vi "TirfModuleStep.vi"() -> ()   [LabVIEW 2012]
doc: "DESCRIPTION:\nThe One-Axis Move (Accel - Max Velocity - Decel) VI completes a move to user-specified position on a single axis while using user-specified acceleration, maximum velocity, and deceleration values. It also provides a monitor to track the progress of the move.\n\n*Note: This VI can be used as a subVI in a higher level program.\n\nINSTRUCTIONS:\n(1) Be sure your board is initialized before running this VI. Refer to the Initialization topic in the FlexMotion VI Online Help, which can be launched by choosing FlexMotion VI Online Help in the Help menu.\n\n(2) Select the Board ID that corresponds to your FlexMotion controller in the Board Configuration Utility. \n\n(3) Select the axis number to be used.\n\n(4) Set the Target Position (in encoder counts) to which you want the axis to move.\n\n(5) Set the values you wish to use for maximum velocity (RPM), acceleration (RPS/S), and deceleration (RPS/S).\n\n(6) Run the VI.\n\nKEY PARAMETERS:\n(1) Target Position: The position to which you want to move. This value needs to be changed every time you run the VI. If you run the VI twice in a row with the same target position, the motor will not move the second time since it will already be at its target position.\n\n(2) Velocity: The maximum velocity for the specified axis during the move.\n\n(3) Acceleration: The acceleration for the axis during the move.\n\n(4) Deceleration: The deceleration for the axis during the move. (This may be different than the acceleration.)\n\nI/O CONNECTIONS OVERVIEW:\nThis example requires a system configuration with one axis."
uses:
  MicroDrive.dll
panel:
  in  "Move This Axis":u16(ring)=1 items=["1"=1, "2"=2, "3"=3, "4"=4, "5"=5, "6"=6]
  out "M6 Forward Limit":bool
  out "M6 Reverse Limit":bool
  out "M5 Forward Limit":bool
  out "M5 Reverse Limit":bool
  out "M4 Forward Limit":bool
  out "M4 Reverse Limit":bool
  in  "Reset M4":bool
  in  "Flip M4 Encoder":bool
  out "M4 Encoder (um)":dbl format="%.3f"
  in  "Flip M3 Encoder":bool
  in  "Flip M2 Encoder":bool
  in  "Flip M1 Encoder":bool
  out "M3 Encoder (um)":dbl format="%.3f"
  in  "Reset M3":bool
  out "M3 Forward Limit":bool
  out "M3 Reverse Limit":bool
  out "M2 Forward Limit":bool
  out "M2 Reverse Limit":bool
  out "M1 Forward Limit":bool
  out "M1 Reverse Limit":bool
  out "M2 Encoder (um)":dbl format="%.3f"
  in  "Reset  All":bool
  in  "Reset M2":bool
  out "M1 Encoder (um)":dbl format="%.3f"
  in  "Reset M1":bool
  out "Found Epi":bool
  in  "EPI Axis":u16(ring)=6 items=["1"=1, "2"=2, "3"=3, "4"=4, "5"=5, "6"=6]
  in  "Load":bool
  in  "Save":bool
  in  "clear5":bool
  in  "clear4":bool
  in  "clear3":bool
  in  "clear2":bool
  in  "clear1":bool
  in  "clear all":bool
  in  "write 5":bool
  in  "write 4":bool
  in  "write 3":bool
  in  "write 2":bool
  in  "write 1":bool
  in  "p4":bool
  in  "p5":bool
  in  "p3":bool
  in  "p2":bool
  in  "p1":bool
  out "Cluster":cluster{"Name":string[], "Position":dbl[]}
  out "Array 2":string[](array[string])
  out "Array":dbl[](array[numeric])
  out "Moving":bool
  in  "EPI":bool
  in  "Store":bool
  out "Current Position":dbl
  in  "Direction:":bool=TRUE
  out "Device Handle":i32
  in  "Velocity (mm/s)":dbl=1.0 min=0.01 max=2.0 format="%.3f"
  in  "Move size (µm)":dbl=50.0 format="%.3f"
  out "Forward Limit":bool
  out "Reverse Limit":bool
  in  "stop":bool
  in  "Move":bool
  # "Move To:"
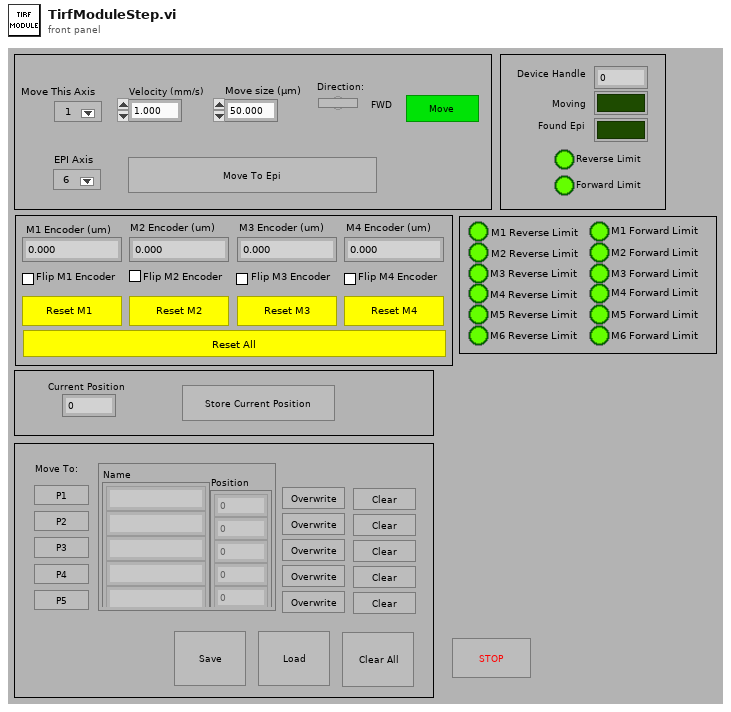
[diagram p1: front panel]
types:
  T1 = enum8{"Enabled", "Disabled", "Disabled and Grayed Out"}
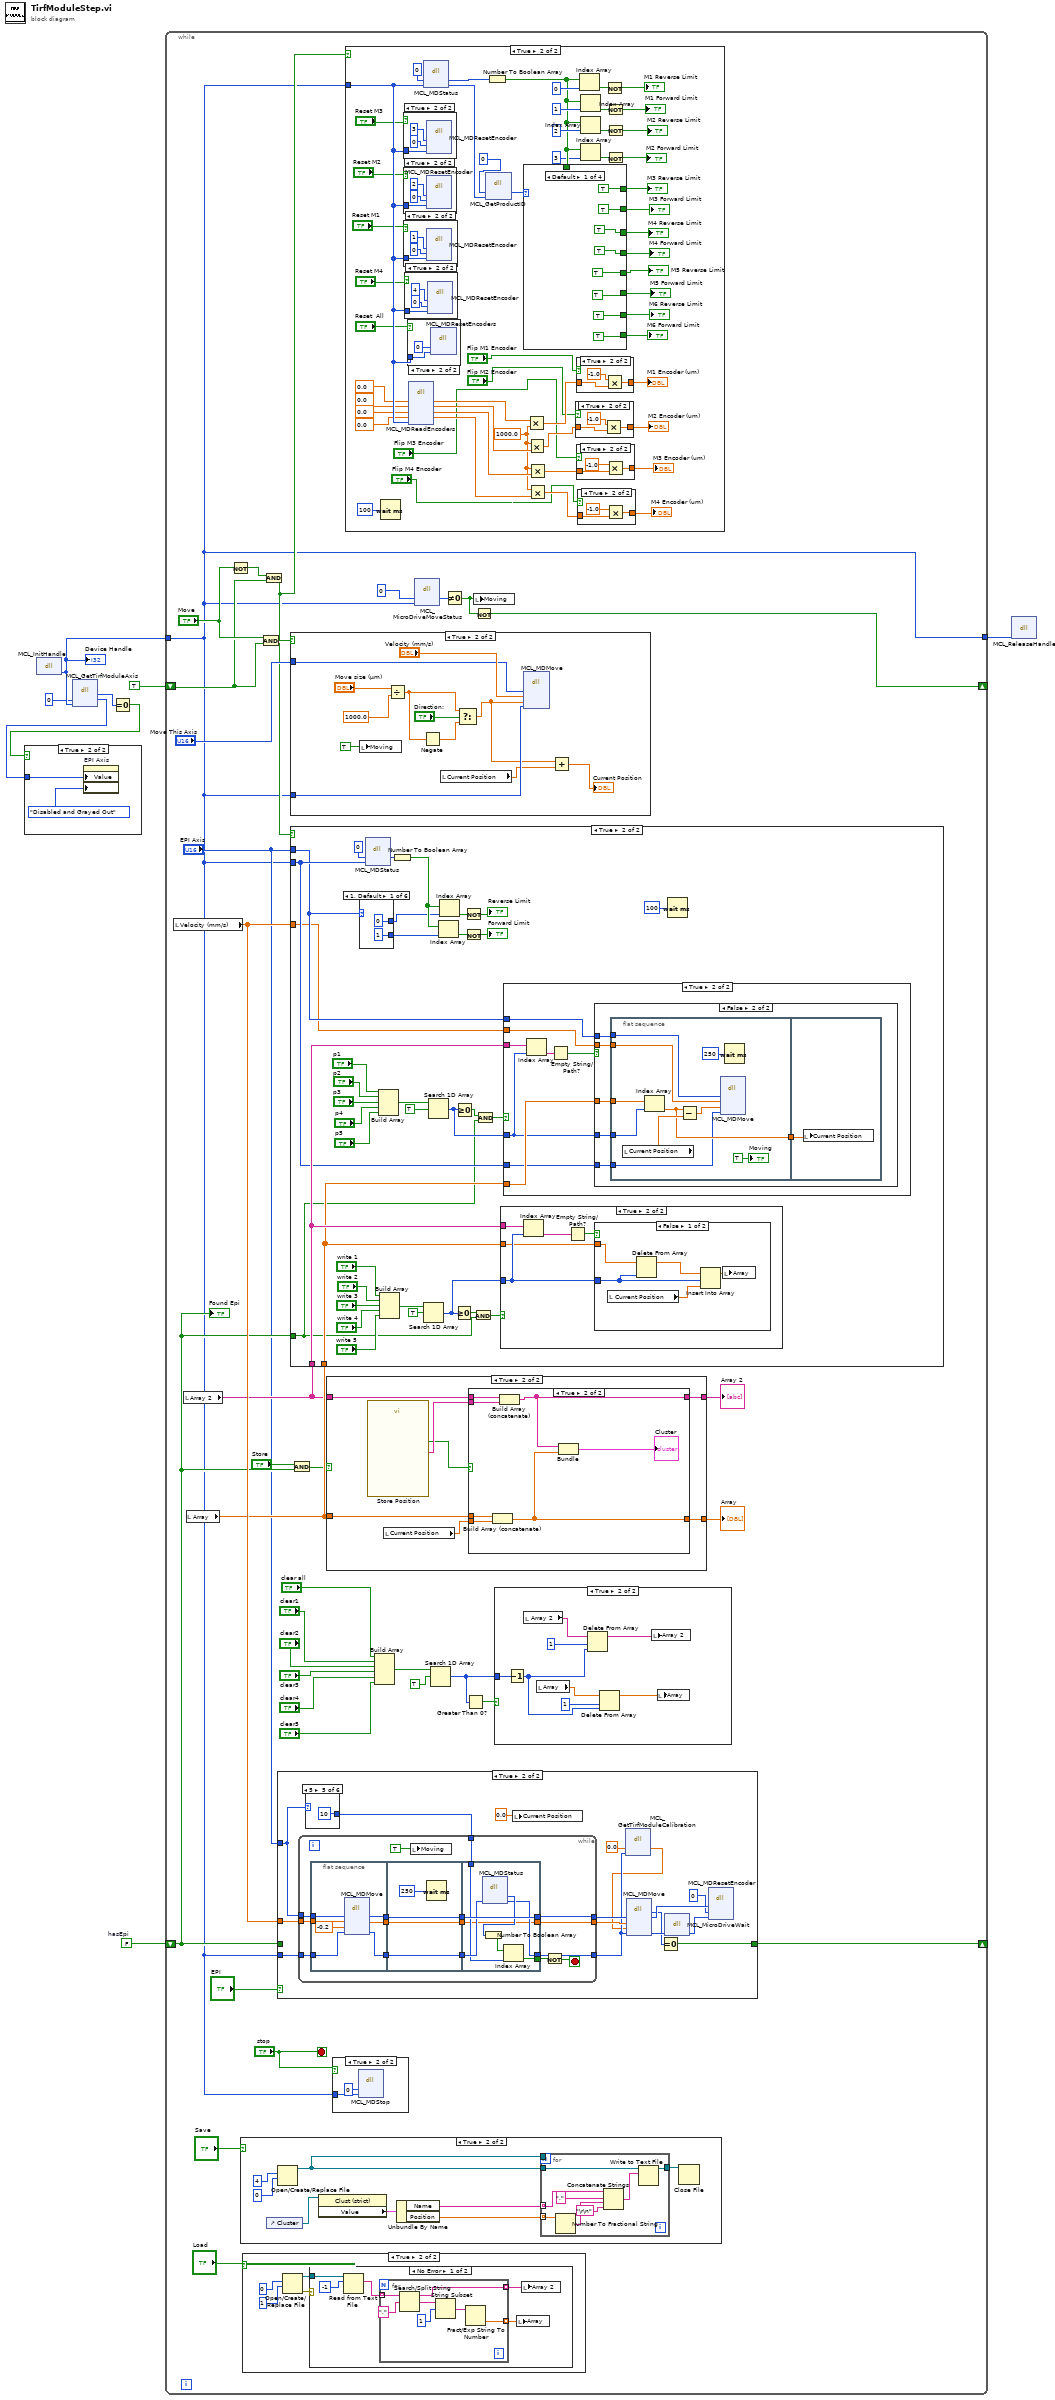
[diagram p0: block diagram]
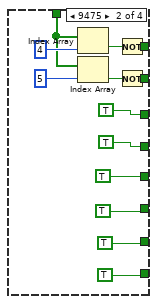
[diagram p9: hidden frame]
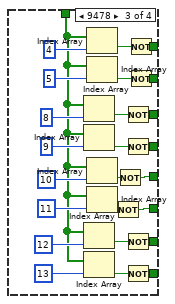
[diagram p10: hidden frame]
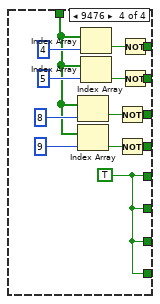
[diagram p11: hidden frame]
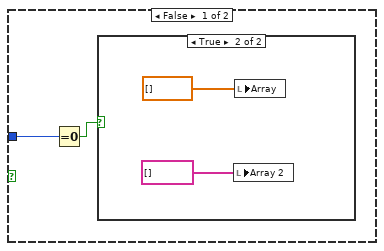
[diagram p19: hidden frame]
diagram:
  w6 = FALSE  # hasEpi
  n1 = dll-call lib="C:/Users/Labview/Desktop/TirfModuleStep/MicroDrive.dll" fn="MCL_InitHandle"() -> ("return type"=w5:i32)  [unwired: 3 in, 2 out]
  "Device Handle" <- w5
  n2 = dll-call lib="C:/Users/Labview/Desktop/TirfModuleStep/MicroDrive.dll" fn="MCL_GetTirfModuleAxis"("axis"=u16 0, "handle"=w5) -> ("return type"=w3:i32, "axis"=w1:i32)  [unwired: 4 in, 2 out]
  n3 = Equal To 0?(x=w3) -> (x = 0?=w2:bool)
  n4 = case shown="True" w2 {
    tunnel: w1 -> [_ w10]
    frame False {
    }
    frame True {
      n5 = property on="EPI Axis" class="Ring (strict)"("Value"=w10, "DisabledEnum"=T1."Disabled and Grayed Out" ("Disabled")) -> ()  [unwired: 2 in, 2 out]
    }
  }
  n6 = while {
    tunnel: w5 -> [w15]
    shift-right: [w12] -> _
    shift-left: TRUE -> [w43]
    tunnel: [w15] -> w7
    shift-right: [w22] -> _
    shift-left: w6 -> [w19]
    stop <- "stop" stop-if-true
    n7 = local read "Velocity (mm/s)"() -> (w40:dbl)
    n8 = local read "Array 2"() -> (w37:string[])
    n9 = local read "Array"() -> (w39:dbl[])
    n10 = Not(x="Move") -> (.not. x?=w44:bool)
    n11 = case shown="True" "Save" {
      frame False {
      }
      frame True {
        n12 = control-ref of="Cluster"() -> (w212:refnum<vi>)
        n13 = Open/Create/Replace File(operation (0:open)=4, access (0:read/write)=0) -> (refnum out=w206:refnum<file>)  [unwired: 4 in, 2 out]
        n14 = property class="Clust (strict)"(reference=w212) -> ("Value"=w211:cluster{"Name":string[], "Position":dbl[]})  [unwired: 1 in, 2 out]
        n15 = Unbundle By Name(w211) -> ("Name"=w207:string[], "Position"=w205:dbl[])
        n16 = for {
          tunnel: w205 -> [w219] mode=indexing
          tunnel: w206 -> [_]
          tunnel: [w220] -> w208
          tunnel: w207 -> [w214] mode=indexing
          tunnel: w206 -> [w213]
          n17 = Number To Fractional String(number=w219) -> (F-format string=w215:string)  [unwired: 3 in]
          n18 = Concatenate Strings(w214, ",", w215, "\r\n") -> (w217:string)
          n19 = Write to Text File(file (use dialog)=w213, text=w217) -> (refnum out=w220:refnum<file>)  [unwired: 2 in, 2 out]
        }
        n20 = Close File(refnum=w208) -> ()  [unwired: 1 in, 2 out]
      }
    }
    n21 = case shown="True" "Load" {
      frame False {
      }
      frame True {
        n22 = Open/Create/Replace File(operation (0:open)=0, access (0:read/write)=1) -> (refnum out=w189:refnum<file>, error out=w190:errorcluster)  [unwired: 4 in, 1 out]
        n23 = case shown="No Error" w190 {
          tunnel: w189 -> [w197 _]
          frame No Error {
            n24 = Read from Text File(file (use dialog)=w197, count=-1) -> (text=w195:string[])  [unwired: 2 in, 3 out]
            n25 = for {
              tunnel: w195 -> [w204] mode=indexing
              tunnel: [w202] -> w194 mode=indexing
              tunnel: [w198] -> w193 mode=indexing
              n26 = Search/Split String(string=w204, search string/char (-)=",") -> (substring before match=w202:string, match + rest of string=w201:string)  [unwired: 1 in, 1 out]
              n27 = String Subset(string=w201, offset (0)=1) -> (substring=w199:string)  [unwired: 1 in]
              n28 = Fract/Exp String To Number(string=w199) -> (number=w198:dbl)  [unwired: 3 in, 1 out]
            }
            n29 = local write "Array"(w193) -> ()
            n30 = local write "Array 2"(w194) -> ()
          }
          frame Error {
          }
        }
      }
    }
    n31 = And(x="Move", y=w43) -> (x .and. y?=w42:bool)
    n32 = And(x=w44, y=w43) -> (x .and. y?=w16:bool)
    n33 = case shown="True" "EPI" {
      tunnel: w40 -> [_ w334]
      tunnel: w15 -> [_ w333]
      tunnel: "EPI Axis" -> [_ w330]
      tunnel: w19 -> [w318 _]
      tunnel: [w318 w319] -> w22
      frame False {
      }
      frame True {
        n34 = case shown="5" w330 {
          tunnel: [0 2 4 8 10 12] -> w329
          frame 1, Default {
          }
          frame 2 {
          }
          frame 3 {
          }
          frame 4 {
          }
          frame 5 {
          }
          frame 6 {
          }
        }
        n35 = while {
          tunnel: w334 -> [w356]
          tunnel: w333 -> [w352]
          tunnel: [w351] -> w322
          tunnel: w330 -> [w354]
          tunnel: [w353] -> w327
          tunnel: w329 -> [w346]
          tunnel: [w342] -> w328
          stop <- w355 stop-if-true
          n36 = flat-sequence {
            tunnel: w356 -> [w363]
            tunnel: w354 -> [w361]
            tunnel: w352 -> [w359]
            tunnel: [w360] -> w350
            tunnel: [w358] -> w349
            tunnel: [w357] -> w344
            tunnel: w350 -> [w367]
            tunnel: w349 -> [w366]
            tunnel: [w367] -> w348
            tunnel: [w366] -> w347
            tunnel: w344 -> [w364]
            tunnel: [w364] -> w343
            tunnel: [w371] -> w351
            tunnel: [w375] -> w353
            tunnel: w348 -> [w375]
            tunnel: w347 -> [w372]
            tunnel: w346 -> [w370]
            tunnel: [w369] -> w345
            tunnel: w343 -> [w368]
            tunnel: [w368] -> w342
            frame #0 {
              n37 = dll-call lib="C:/Users/Labview/Desktop/TirfModuleStep/MicroDrive.dll" fn="MCL_MDMove"("axis"=w361, "velocity"=w363, "distance"=-0.2, "handle"=w359) -> ("axis"=w360:i32, "velocity"=w357:dbl, "handle"=w358:i32)  [unwired: 4 in, 3 out]
            }
            frame #1 {
              n38 = Wait (ms)(milliseconds to wait=u32 250) -> ()  [unwired: 1 out]
            }
            frame #2 {
              n39 = dll-call lib="C:/Users/Labview/Desktop/TirfModuleStep/MicroDrive.dll" fn="MCL_MDStatus"("handle"=w372) -> ("status"=w374:u16, "handle"=w371:i32)  [unwired: 3 in, 4 out]
              n40 = Number To Boolean Array(number=w374) -> (Boolean array=w373:bool[])
              n41 = Index Array(array=w373, index=w370) -> (element=w369:bool)
            }
          }
          n42 = local write "Moving"(TRUE ("is Moving")) -> ()
          n43 = Not(x=w345) -> (.not. x?=w355:bool)
        }
        n44 = local write "Current Position"(0.0) -> ()
        n45 = dll-call lib="C:/Users/Labview/Desktop/TirfModuleStep/MicroDrive.dll" fn="MCL_GetTirfModuleCalibration"("calMM"=0.0 ("distance"), "handle"=w322) -> ("calMM"=w321:dbl)  [unwired: 4 in, 3 out]
        n46 = dll-call lib="C:/Users/Labview/Desktop/TirfModuleStep/MicroDrive.dll" fn="MCL_MDMove"("axis"=w327, "velocity"=w328, "distance"=w321, "handle"=w322) -> ("return type"=w320:i32, "axis"=w325:i32, "handle"=w331:i32)  [unwired: 5 in, 2 out]
        n47 = Equal To 0?(x=w320) -> (x = 0?=w319:bool)
        n48 = dll-call lib="C:/Users/Labview/Desktop/TirfModuleStep/MicroDrive.dll" fn="MCL_MicroDriveWait"("handle"=w331) -> ("handle"=w326:i32)  [unwired: 3 in, 3 out]
        n49 = dll-call lib="C:/Users/Labview/Desktop/TirfModuleStep/MicroDrive.dll" fn="MCL_MDResetEncoder"("axis"=w325, "status"=u16 0 ("distance"), "handle"=w326) -> ()  [unwired: 5 in, 4 out]
      }
    }
    n50 = case shown="True" w42 {
      tunnel: w15 -> [_ w405]
      tunnel: "Move This Axis" -> [_ w397]
      frame False {
      }
      frame True {
        n51 = local write "Moving"(TRUE ("is Moving")) -> ()
        n52 = Divide(x="Move size (µm)", y=1000.0) -> (x/y=w402:dbl)
        n53 = Negate(x=w402) -> (-x=w403:dbl)
        n54 = local read "Current Position"() -> (w399:dbl)
        n55 = Select(t=w402, s="Direction:", f=w403) -> (s? t:f=w401:dbl)
        n56 = dll-call lib="C:/Users/Labview/Desktop/TirfModuleStep/MicroDrive.dll" fn="MCL_MDMove"("axis"=w397, "velocity"="Velocity (mm/s)", "distance"=w401, "handle"=w405) -> ()  [unwired: 6 in, 4 out]
        n57 = Add(x=w401, y=w399) -> (x+y=→"Current Position":dbl)
      }
    }
    n58 = case shown="True" w16 {
      tunnel: w37 -> [_ w268]
      tunnel: w40 -> [_ w238]
      tunnel: w39 -> [_ w267]
      tunnel: "EPI Axis" -> [_ w239]
      tunnel: w15 -> [_ w240]
      tunnel: w19 -> [_ w234]
      frame False {
      }
      frame True {
        n59 = case shown="1, Default" w239 {
          tunnel: [0 2 4 8 10 12] -> w242
          tunnel: [1 3 5 9 11 13] -> w241
          frame 1, Default {
          }
          frame 2 {
          }
          frame 3 {
          }
          frame 4 {
          }
          frame 5 {
          }
          frame 6 {
          }
        }
        n60 = dll-call lib="C:/Users/Labview/Desktop/TirfModuleStep/MicroDrive.dll" fn="MCL_MDStatus"("status"=u16 0, "handle"=w240) -> ("status"=w264:u16)  [unwired: 4 in, 3 out]
        n61 = Build Array("p1", "p2", "p3", "p4", "p5") -> (w249:bool[])
        n62 = Build Array("write 1", "write 2", "write 3", "write 4", "write 5") -> (w257:bool[])
        n63 = Number To Boolean Array(number=w264) -> (Boolean array=w263:bool[])
        n64 = Search 1D Array(1D array=w257, element=TRUE) -> (index of element=w256:i32)  [unwired: 1 in]
        n65 = Search 1D Array(1D array=w249, element=TRUE) -> (index of element=w243:i32)  [unwired: 1 in]
        n66 = Index Array(array=w263, index=w241) -> (element=w262:bool)
        n67 = Index Array(array=w263, index=w242) -> (element=w261:bool)
        n68 = Greater Or Equal To 0?(x=w256) -> (x >= 0?=w237:bool)
        n69 = Greater Or Equal To 0?(x=w243) -> (x >= 0?=w233:bool)
        n70 = Not(x=w261) -> (.not. x?=→"Reverse Limit":bool)
        n71 = Not(x=w262) -> (.not. x?=→"Forward Limit":bool)
        n72 = And(x=w237, y=w234) -> (x .and. y?=w236:bool)
        n73 = And(x=w233, y=w234) -> (x .and. y?=w235:bool)
        n74 = case shown="True" w236 {
          tunnel: w268 -> [_ w285]
          tunnel: w267 -> [_ w281]
          tunnel: w256 -> [_ w282]
          frame False {
          }
          frame True {
            n75 = Index Array(array=w285, index=w282) -> (element=w284:string)
            n76 = Empty String/Path?(string/path=w284) -> (empty?=w283:bool)
            n77 = case shown="False" w283 {
              tunnel: w282 -> [w289 _]
              tunnel: w281 -> [w286 _]
              frame False {
                n78 = local read "Current Position"() -> (w288:dbl)
                n79 = Delete From Array(array=w286, index=w289) -> (array with subset deleted=w290:dbl[])  [unwired: 1 in, 1 out]
                n80 = Insert Into Array(array=w290, index=w289, new element=w288) -> (w287:dbl[])
                n81 = local write "Array"(w287) -> ()
              }
              frame True {
                n82 = One Button Dialog(message="This position is not defined.") -> ()  [unwired: 1 in, 1 out]
              }
            }
          }
        }
        n83 = case shown="True" w235 {
          tunnel: w267 -> [_ w299]
          tunnel: w240 -> [_ w298]
          tunnel: w238 -> [_ w297]
          tunnel: w268 -> [_ w296]
          tunnel: w243 -> [_ w293]
          tunnel: w239 -> [_ w292]
          frame False {
          }
          frame True {
            n84 = Index Array(array=w296, index=w293) -> (element=w295:string)
            n85 = Empty String/Path?(string/path=w295) -> (empty?=w294:bool)
            n86 = case shown="False" w294 {
              tunnel: w299 -> [_ w306]
              tunnel: w298 -> [_ w305]
              tunnel: w297 -> [_ w304]
              tunnel: w293 -> [_ w303]
              tunnel: w292 -> [_ w301]
              frame True {
                n87 = One Button Dialog(message="This position is not defined.") -> ()  [unwired: 1 in, 1 out]
              }
              frame False {
                n88 = flat-sequence {
                  tunnel: w306 -> [w316]
                  tunnel: w305 -> [w309]
                  tunnel: w304 -> [w308]
                  tunnel: w303 -> [w312]
                  tunnel: [w310] -> w302
                  tunnel: w301 -> [w307]
                  tunnel: w302 -> [w317]
                  frame #0 {
                    n89 = local read "Current Position"() -> (w314:dbl)
                    n90 = Index Array(array=w316, index=w312) -> (element=w310:dbl)
                    n91 = Subtract(x=w310, y=w314) -> (x-y=w315:dbl)
                    n92 = dll-call lib="C:/Users/Labview/Desktop/TirfModuleStep/MicroDrive.dll" fn="MCL_MDMove"("axis"=w307, "velocity"=w308, "distance"=w315, "handle"=w309) -> ()  [unwired: 6 in, 4 out]
                    n93 = Wait (ms)(milliseconds to wait=u32 250) -> ()  [unwired: 1 out]
                    "Moving" <- TRUE ("is Moving")
                  }
                  frame #1 {
                    n94 = local write "Current Position"(w317) -> ()
                  }
                }
              }
            }
          }
        }
        n95 = Wait (ms)(milliseconds to wait=100) -> ()  [unwired: 1 out]
      }
    }
    n96 = And(x="Store", y=w19) -> (x .and. y?=w20:bool)
    n97 = case shown="True" w20 {
      tunnel: w37 -> [w378 w385]
      tunnel: [w378 w381] -> w36
      tunnel: w39 -> [w376 w384]
      tunnel: [w376 w380] -> w38
      frame False {
        n98 = Bundle("Array 2"=w378, "Array"=w376) -> (w377:cluster{"Array 2":string[], "Array":dbl[]})  [unwired: 1 in]
        n99 = local write "Cluster"(w377) -> ()
      }
      frame True {
        n100 = call "Store Position"() -> ("Name"=w383:string, "OK"=w379:bool)  [unwired: 17 in, 1 out]
        n101 = local read "Current Position"() -> (w382:dbl)
        n102 = case shown="True" w379 {
          tunnel: w385 -> [w387 w394]
          tunnel: w384 -> [w386 w393]
          tunnel: w383 -> [_ w392]
          tunnel: w382 -> [_ w391]
          tunnel: [w387 w390] -> w381
          tunnel: [w386 w388] -> w380
          frame False {
          }
          frame True {
            n103 = Build Array (concatenate)(w393, w391) -> (w388:dbl[])
            n104 = Build Array (concatenate)(w394, w392) -> (w390:string[])
            n105 = Bundle(w390, w388) -> (→"Cluster":cluster{string[], dbl[]})  [unwired: 1 in]
          }
        }
      }
    }
    "Array" <- w38
    "Array 2" <- w36
    n106 = case shown="True" "stop" {
      tunnel: w15 -> [_ w395]
      frame False {
      }
      frame True {
        n107 = dll-call lib="C:/Users/Labview/Desktop/TirfModuleStep/MicroDrive.dll" fn="MCL_MDStop"("status"=0, "handle"=w395) -> ()  [unwired: 4 in, 4 out]
      }
    }
    n108 = case shown="True" w16 {
      tunnel: w15 -> [_ w89]
      frame False {
      }
      frame True {
        w77 = 1000.0
        n109 = Wait (ms)(milliseconds to wait=100) -> ()  [unwired: 1 out]
        n110 = case shown="True" "Reset M3" {
          tunnel: w89 -> [_ w101]
          frame False {
          }
          frame True {
            n111 = dll-call lib="C:/Users/Labview/Desktop/TirfModuleStep/MicroDrive.dll" fn="MCL_MDResetEncoder"("axis"=u32 3, "status"=u16 0, "handle"=w101) -> ()  [unwired: 4 in, 5 out]
          }
        }
        n112 = case shown="True" "Reset M2" {
          tunnel: w89 -> [_ w104]
          frame False {
          }
          frame True {
            n113 = dll-call lib="C:/Users/Labview/Desktop/TirfModuleStep/MicroDrive.dll" fn="MCL_MDResetEncoder"("axis"=u32 2, "status"=u16 0, "handle"=w104) -> ()  [unwired: 4 in, 5 out]
          }
        }
        n114 = case shown="True" "Reset M1" {
          tunnel: w89 -> [_ w107]
          frame False {
          }
          frame True {
            n115 = dll-call lib="C:/Users/Labview/Desktop/TirfModuleStep/MicroDrive.dll" fn="MCL_MDResetEncoder"("axis"=u32 1, "status"=u16 0, "handle"=w107) -> ()  [unwired: 4 in, 5 out]
          }
        }
        n116 = case shown="True" "Reset M4" {
          tunnel: w89 -> [_ w110]
          frame False {
          }
          frame True {
            n117 = dll-call lib="C:/Users/Labview/Desktop/TirfModuleStep/MicroDrive.dll" fn="MCL_MDResetEncoder"("axis"=u32 4, "status"=u16 0, "handle"=w110) -> ()  [unwired: 4 in, 5 out]
          }
        }
        n118 = case shown="True" "Reset  All" {
          tunnel: w89 -> [_ w112]
          frame False {
          }
          frame True {
            n119 = dll-call lib="C:/Users/Labview/Desktop/TirfModuleStep/MicroDrive.dll" fn="MCL_MDResetEncoders"("status"=u16 0, "handle"=w112) -> ()  [unwired: 4 in, 4 out]
          }
        }
        n120 = dll-call lib="C:/Users/Labview/Desktop/TirfModuleStep/MicroDrive.dll" fn="MCL_MDReadEncoders"("m1"=0.0, "m2"=0.0, "m3"=0.0, "m4"=0.0, "handle"=w89) -> ("m1"=w87:dbl, "m2"=w86:dbl, "m3"=w85:dbl, "m4"=w88:dbl)  [unwired: 4 in, 3 out]
        n121 = dll-call lib="C:/Users/Labview/Desktop/TirfModuleStep/MicroDrive.dll" fn="MCL_MDStatus"("status"=u16 0, "handle"=w89) -> ("status"=w84:u16)  [unwired: 4 in, 3 out]
        n122 = dll-call lib="C:/Users/Labview/Desktop/TirfModuleStep/MicroDrive.dll" fn="MCL_GetProductID"("PID"=u16 0, "handle"=w89) -> ("PID"=w78:u16)  [unwired: 4 in, 3 out]
        n123 = Number To Boolean Array(number=w84) -> (Boolean array=w90:bool[])
        n124 = case shown="Default" w78 {
          tunnel: [TRUE w132 w157 w171] -> w65
          tunnel: w90 -> [_ w130 w134 w160]
          tunnel: [TRUE w128 w154 w168] -> w66
          tunnel: [TRUE TRUE w140 w162] -> w64
          tunnel: [TRUE TRUE w139 w161] -> w59
          tunnel: [TRUE TRUE w138 w159] -> w60
          tunnel: [TRUE TRUE w137 w159] -> w61
          tunnel: [TRUE TRUE w136 w159] -> w63
          tunnel: [TRUE TRUE w135 w159] -> w62
          frame Default {
          }
          frame 9475 {
            n125 = Index Array(array=w130, index=4) -> (element=w133:bool)
            n126 = Index Array(array=w130, index=5) -> (element=w127:bool)
            n127 = Not(x=w133) -> (.not. x?=w132:bool)
            n128 = Not(x=w127) -> (.not. x?=w128:bool)
          }
          frame 9478 {
            n129 = Index Array(array=w134, index=8) -> (element=w152:bool)
            n130 = Index Array(array=w134, index=9) -> (element=w149:bool)
            n131 = Index Array(array=w134, index=12) -> (element=w144:bool)
            n132 = Index Array(array=w134, index=13) -> (element=w141:bool)
            n133 = Index Array(array=w134, index=4) -> (element=w158:bool)
            n134 = Index Array(array=w134, index=5) -> (element=w153:bool)
            n135 = Index Array(array=w134, index=10) -> (element=w148:bool)
            n136 = Index Array(array=w134, index=11) -> (element=w145:bool)
            n137 = Not(x=w145) -> (.not. x?=w137:bool)
            n138 = Not(x=w148) -> (.not. x?=w138:bool)
            n139 = Not(x=w152) -> (.not. x?=w140:bool)
            n140 = Not(x=w149) -> (.not. x?=w139:bool)
            n141 = Not(x=w144) -> (.not. x?=w136:bool)
            n142 = Not(x=w141) -> (.not. x?=w135:bool)
            n143 = Not(x=w158) -> (.not. x?=w157:bool)
            n144 = Not(x=w153) -> (.not. x?=w154:bool)
          }
          frame 9476 {
            w159 = TRUE
            n145 = Index Array(array=w160, index=8) -> (element=w166:bool)
            n146 = Index Array(array=w160, index=9) -> (element=w163:bool)
            n147 = Index Array(array=w160, index=4) -> (element=w172:bool)
            n148 = Index Array(array=w160, index=5) -> (element=w167:bool)
            n149 = Not(x=w166) -> (.not. x?=w162:bool)
            n150 = Not(x=w163) -> (.not. x?=w161:bool)
            n151 = Not(x=w172) -> (.not. x?=w171:bool)
            n152 = Not(x=w167) -> (.not. x?=w168:bool)
          }
        }
        "M4 Reverse Limit" <- w64
        "M3 Forward Limit" <- w66
        "M3 Reverse Limit" <- w65
        "M5 Reverse Limit" <- w60
        "M5 Forward Limit" <- w61
        "M6 Reverse Limit" <- w63
        "M6 Forward Limit" <- w62
        "M4 Forward Limit" <- w59
        n153 = Multiply(x=w87, y=w77) -> (x*y=w79:dbl)
        n154 = Multiply(x=w77, y=w86) -> (x*y=w80:dbl)
        n155 = Multiply(x=w77, y=w85) -> (x*y=w81:dbl)
        n156 = Multiply(x=w77, y=w88) -> (x*y=w76:dbl)
        n157 = case shown="True" "Flip M2 Encoder" {
          tunnel: w80 -> [w177 w179]
          tunnel: [w177 w180] -> w52
          frame False {
          }
          frame True {
            n158 = Multiply(x=-1.0, y=w179) -> (x*y=w180:dbl)
          }
        }
        "M2 Encoder (um)" <- w52
        n159 = case shown="True" "Flip M1 Encoder" {
          tunnel: w79 -> [w173 w175]
          tunnel: [w173 w176] -> w49
          frame False {
          }
          frame True {
            n160 = Multiply(x=-1.0, y=w175) -> (x*y=w176:dbl)
          }
        }
        "M1 Encoder (um)" <- w49
        n161 = case shown="True" "Flip M3 Encoder" {
          tunnel: w81 -> [w181 w183]
          tunnel: [w181 w184] -> w50
          frame False {
          }
          frame True {
            n162 = Multiply(x=-1.0, y=w183) -> (x*y=w184:dbl)
          }
        }
        "M3 Encoder (um)" <- w50
        n163 = case shown="True" "Flip M4 Encoder" {
          tunnel: w76 -> [w185 w187]
          tunnel: [w185 w188] -> w51
          frame False {
          }
          frame True {
            n164 = Multiply(x=-1.0, y=w187) -> (x*y=w188:dbl)
          }
        }
        "M4 Encoder (um)" <- w51
        n165 = Index Array(array=w90, index=0) -> (element=w91:bool)
        n166 = Index Array(array=w90, index=1) -> (element=w92:bool)
        n167 = Index Array(array=w90, index=2) -> (element=w93:bool)
        n168 = Index Array(array=w90, index=3) -> (element=w82:bool)
        n169 = Not(x=w91) -> (.not. x?=→"M1 Reverse Limit":bool)
        n170 = Not(x=w92) -> (.not. x?=→"M1 Forward Limit":bool)
        n171 = Not(x=w93) -> (.not. x?=→"M2 Reverse Limit":bool)
        n172 = Not(x=w82) -> (.not. x?=→"M2 Forward Limit":bool)
      }
    }
    n173 = Build Array("clear all", "clear1", "clear2", "clear3", "clear4", "clear5") -> (w29:bool[])
    n174 = dll-call lib="C:/Users/Labview/Desktop/TirfModuleStep/MicroDrive.dll" fn="MCL_MicroDriveMoveStatus"("isMoving"=u16 0, "handle"=w15) -> ("isMoving"=w14:i32)  [unwired: 4 in, 3 out]
    n175 = Search 1D Array(1D array=w29, element=TRUE) -> (index of element=w28:i32)  [unwired: 1 in]
    n176 = Not Equal To 0?(x=w14) -> (x != 0?=w13:bool)
    n177 = Greater Than 0?(x=w28) -> (x > 0?=w30:bool)
    n178 = local write "Moving"(w13) -> ()
    n179 = Not(x=w13) -> (.not. x?=w12:bool)
    n180 = case shown="True" w30 {
      tunnel: w28 -> [w222 w228]
      frame False {
        n181 = Equal To 0?(x=w222) -> (x = 0?=w221:bool)
        n182 = case shown="True" w221 {
          frame False {
          }
          frame True {
            n183 = local write "Array 2"(string[] []) -> ()
            n184 = local write "Array"(dbl[] []) -> ()
          }
        }
      }
      frame True {
        n185 = Decrement(x=w228) -> (x-1=w225:i32)
        n186 = local read "Array 2"() -> (w230:string[])
        n187 = local read "Array"() -> (w229:dbl[])
        n188 = Delete From Array(array=w230, length=1, index=w225) -> (array with subset deleted=w227:string[])  [unwired: 1 out]
        n189 = Delete From Array(array=w229, length=1, index=w225) -> (array with subset deleted=w226:dbl[])  [unwired: 1 out]
        n190 = local write "Array 2"(w227) -> ()
        n191 = local write "Array"(w226) -> ()
      }
    }
    "Found Epi" <- w19
  }
  n192 = dll-call lib="C:/Users/Labview/Desktop/TirfModuleStep/MicroDrive.dll" fn="MCL_ReleaseHandle"("handle"=w7) -> ()  [unwired: 4 in, 3 out]
